vi "Get Next Empty Cell.vi"(8 "error in (no error)":errorcluster, 11 "MS-Excel in":refnum<class "MS-Excel.lvclass">) -> (0 "error out":errorcluster, 2 "Next Empty Cell":cluster{"Row":i32, "Column":i32}, 3 "MS-Excel out":refnum<class "MS-Excel.lvclass">)   [LabVIEW 2020, in "LabVIEW NPOI.lvlib" / "MS-Excel.lvclass"]
doc: "Returns the position , in <b>Next Empty Cell</b>,of the last cell contained <b>PLUS ONE</b> in the active worksheet of the associated workbook to the <b>Document</b>."
uses:
  MS-Excel.lvclass
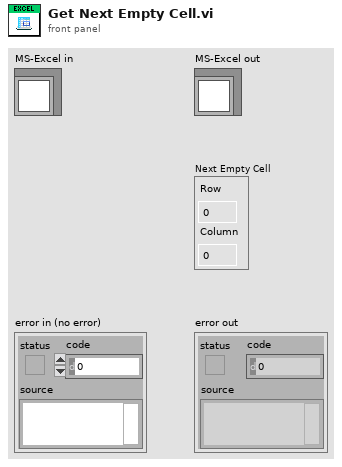
[diagram p1: front panel]
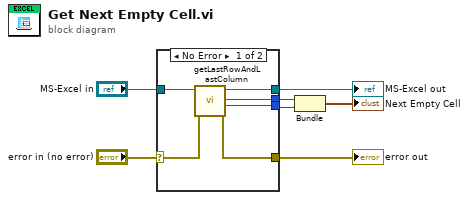
[diagram p0: block diagram]
diagram:
  n1 = case shown="No Error" "error in (no error)" {
    selector: "error in (no error)" -> [w11 w15]
    tunnel: [w10 w15] -> w6
    tunnel: [w12 w14] -> w4
    tunnel: "MS-Excel in" -> [w13 w14]
    tunnel: [w9 _] -> w3
    tunnel: [w8 _] -> w2
    frame No Error {
      n2 = call-dynamic "getLastRowAndLastColumn.vi"("error in (no error)"=w11, "MS-Excel in"=w13) -> ("error out"=w10:errorcluster, "Last Column"=w8:i32, "Last Row"=w9:i32, "MS-Excel out"=w12:refnum<class "MS-Excel.lvclass">)  [unwired: 6 in]
    }
    frame Error {
    }
  }
  "error out" <- w6
  "MS-Excel out" <- w4
  n3 = Bundle("Last Row"=w3, "Last Column"=w2) -> (→"Next Empty Cell":cluster{"Last Row":i32, "Last Column":i32})  [unwired: 1 in]
